vi "rawDataFormated.vi"(1 "Channel Type":T1, 2 "Channel Name":string, 3 "2D Data":dbl[][](array[numeric]), 4 "Non-Uniform Data":T2[](array[typedef])) -> (0 "Non-Uniform Data Output":T2[](array[typedef]))   [LabVIEW 2017]
uses:
  Controls/chanData.ctl
  Controls/chanType.ctl
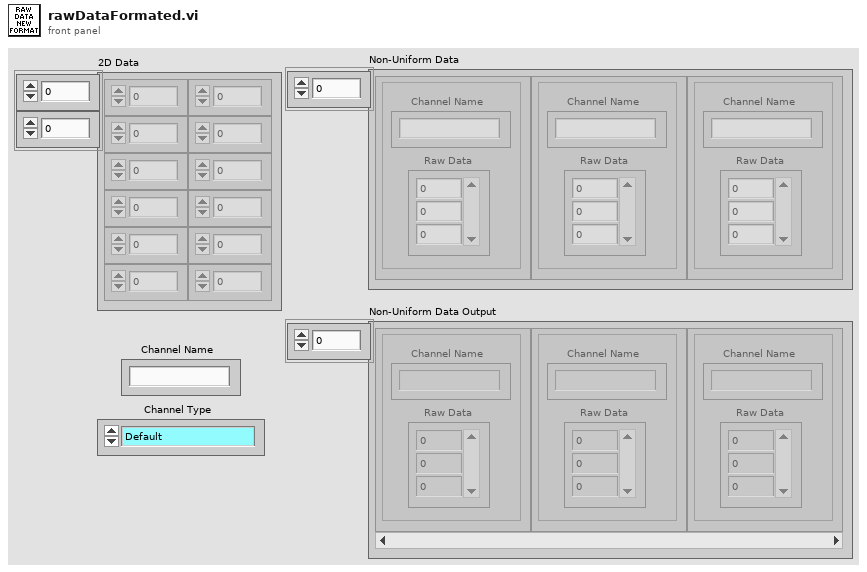
[diagram p1: front panel]
types:
  T1 = typedef "chanType.ctl" = enum16{"Default", "Clock", "Pressure Scanner"}
  T2 = typedef "chanData.ctl" = cluster{"Raw Data":dbl[], "Channel Name":string}
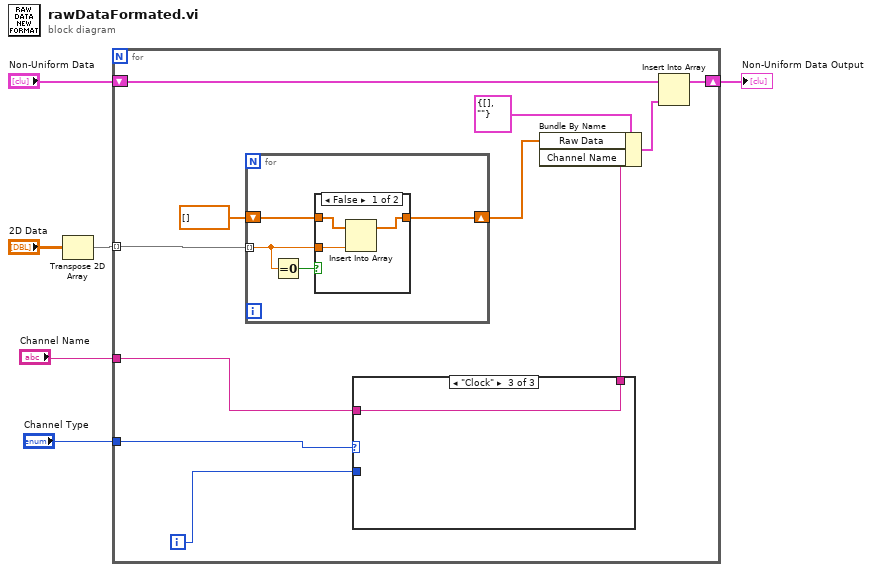
[diagram p0: block diagram]
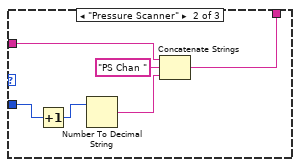
[diagram p3: hidden frame]
diagram:
  n1 = Transpose 2D Array(2D array="2D Data") -> (transposed array=w5:dbl[][])
  n2 = for {
    tunnel: w5 -> [w17] mode=indexing
    shift-right: [w11] -> w1
    shift-left: "Non-Uniform Data" -> [w13]
    tunnel: "Channel Name" -> [w10]
    tunnel: "Channel Type" -> [w7]
    i -> [w8]
    n3 = for {
      tunnel: w17 -> [w28] mode=indexing
      shift-right: [w26] -> w14
      shift-left: dbl[] [] ("array") -> [w27]
      n4 = Equal To 0?(x=w28) -> (x = 0?=w29:bool)
      n5 = case shown="False" w29 {
        tunnel: w28 -> [w32 _]
        tunnel: w27 -> [w31 w33]
        tunnel: [w30 w33] -> w26
        frame False {
          n6 = Insert Into Array(array=w31, new element=w32) -> (w30:dbl[])  [unwired: 1 in]
        }
        frame True {
        }
      }
    }
    n7 = case shown="\"Clock\"" w7 {
      tunnel: w10 -> [w18 w21 w25]
      tunnel: [w18 w22 w25] -> w9
      tunnel: w8 -> [_ w20 _]
      frame "Default", Default {
      }
      frame "Pressure Scanner" {
        n8 = Increment(x=w20) -> (x+1=w19:i32)
        n9 = Number To Decimal String(number=w19) -> (decimal integer string=w23:string)  [unwired: 1 in]
        n10 = Concatenate Strings(w21, "PS Chan " ("string"), w23) -> (w22:string)
      }
      frame "Clock" {
      }
    }
    n11 = Bundle By Name(cluster=T2 {"Raw Data"=[], "Channel Name"=""} ("Channel Data"), "Raw Data"=w14, "Channel Name"=w9) -> (w12:T2)
    n12 = Insert Into Array(array=w13, new element=w12) -> (w11:T2[])  [unwired: 1 in]
  }
  "Non-Uniform Data Output" <- w1
